vi "算法优化模块.vi"(0 "优化算法":u16(ring) items=["无优化", "归一化", "差分算法", "去燥", "对应算法"], 1 "散斑矩阵":dbl[][](array[numeric]), 2 "光源行数":dbl, 3 "图像一维数组":dbl[](array[numeric]), 5 "少量采样数据量M":i32) -> (14 "正图像筛选门限":dbl)   [LabVIEW 2018]
panel:
  # "差分算法输入输出"
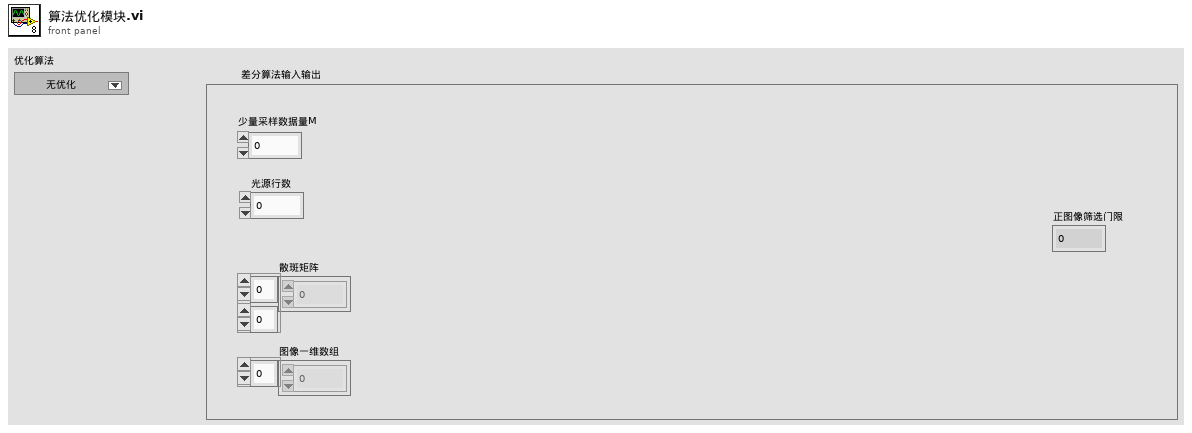
[diagram p1: front panel]
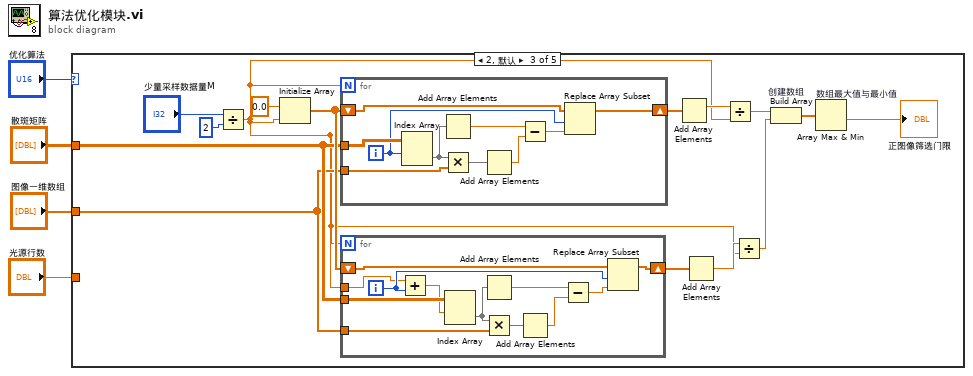
[diagram p0: block diagram]
diagram:
  n1 = case shown="2, 默认" "优化算法" {
    tunnel: "图像一维数组" -> [_ _ w8 _ _]
    tunnel: "散斑矩阵" -> [_ _ w9 _ _]
    tunnel: "光源行数" -> [_ _ _ _ _]
    frame ..0 {
    }
    frame 1 {
    }
    frame 2, Default {
      n2 = Divide(x="少量采样数据量M", y=2) -> (x/y=w6:dbl)
      n3 = Initialize Array(0.0 ("元素"), w6) -> (w10:dbl[])
      n4 = for "For循环" {
        N: w6 -> [_]
        tunnel: w9 -> [w41]
        tunnel: w8 -> [w32]
        shift-right: [w33] -> w17
        shift-left: w10 -> [w36]
        i -> [w34]
        n5 = Index Array(array=w41, index (row)=w34) -> (element=w39:dbl[])  [unwired: 1 in]
        n6 = Add Array Elements(numeric array=w39) -> (sum=w37:dbl)
        n7 = Multiply(x=w39, y=w32) -> (x*y=w40:dbl[])
        n8 = Add Array Elements(numeric array=w40) -> (sum=w38:dbl)
        n9 = Subtract(x=w37, y=w38) -> (x-y=w35:dbl)
        n10 = Replace Array Subset(array=w36, new element=w35, index=w34) -> (w33:dbl[])
      }
      n11 = for {
        N: w6 -> [_]
        tunnel: w9 -> [w31]
        shift-right: [w24] -> w15
        shift-left: w10 -> [w26]
        tunnel: w8 -> [w21]
        tunnel: w6 -> [w20]
        i -> [w22]
        n12 = Add(x=w20, y=w22) -> (x+y=w23:dbl)
        n13 = Index Array(array=w31, index (row)=w23) -> (element=w29:dbl[])  [unwired: 1 in]
        n14 = Add Array Elements(numeric array=w29) -> (sum=w27:dbl)
        n15 = Multiply(x=w29, y=w21) -> (x*y=w30:dbl[])
        n16 = Add Array Elements(numeric array=w30) -> (sum=w28:dbl)
        n17 = Subtract(x=w27, y=w28) -> (x-y=w25:dbl)
        n18 = Replace Array Subset(array=w26, new element=w25, index=w22) -> (w24:dbl[])
      }
      n19 = Add Array Elements(numeric array=w17) -> (sum=w16:dbl)
      n20 = Add Array Elements(numeric array=w15) -> (sum=w14:dbl)
      n21 = Divide(x=w16, y=w6) -> (x/y=w12:dbl)
      n22 = Divide(x=w14, y=w6) -> (x/y=w11:dbl)
      n23 = Build Array "创建数组"(w12, w11) -> (w13:dbl[])
      n24 = Array Max & Min "数组最大值与最小值"(array=w13) -> (min value=→"正图像筛选门限":dbl)  [unwired: 3 out]
    }
    frame 3 {
    }
    frame 4 {
    }
  }
